vi "Project TMP36.vi"() -> ()   [LabVIEW 2023]
uses:
  <vilib>/MakerHub/LINX/Public/Peripherals/PWM/PWM Set Duty Cycle 1 Chan.vi
  <vilib>/MakerHub/LINX/Public/Utilities/Open Serial.vi
  <vilib>/addons/control/pid/pid.llb/PID (DBL).vi
  <vilib>/MakerHub/LINX/Public/Peripherals/PWM/PWM Set Duty Cycle N Chans.vi
  <vilib>/MakerHub/LINX/Public/Sensors/Temperature/TMP3x/TMP36.vi
  <vilib>/addons/control/pid/NI_PID_pid.lvlib
  <vilib>/MakerHub/LINX/LMH-LINX.lvlib
  <vilib>/MakerHub/LINX/Public/Sensors/Temperature/TMP3x/TMP3x.lvlib
panel:
  in  "LowPass Filter\nTf = x Ts":dbl
  out "u":dbl format="%_2f V"
  out "Tout":dbl format="%_4f °C"
  in  "Ts":dbl
  out "Waveform Chart":dbl(graph)
  in  "Initial Value":dbl
  in  "Set Point":dbl
  in  "Stop Button":bool
  in  "PID Controller":cluster{"Kp":dbl, "Ti":dbl, "Td":dbl}
  # "Temperature"
  # "Time"
  # "PID Control"
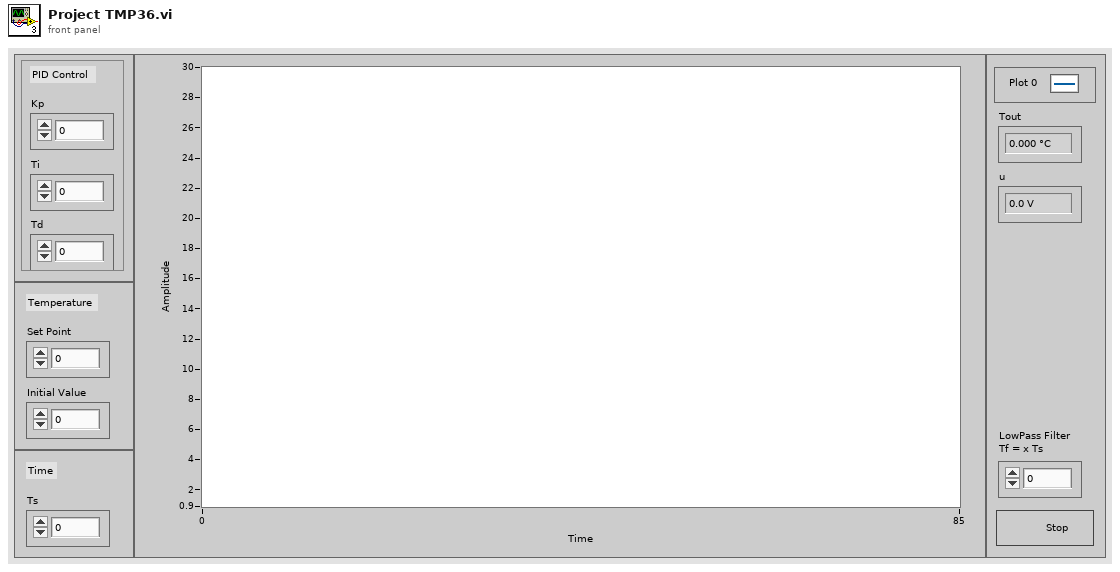
[diagram p1: front panel]
types:
  T1 = typedef "LMH-LINX.lvlib/LINX Ref.ctl" = cluster{"IO":T2, "Interface":T3, "LINX Device Config":T4}
  T2 = typedef "LMH-LINX.lvlib/Platform.ctl" = enum16{"Remote", "Local"}
  T3 = typedef "LMH-LINX.lvlib/Interface.ctl" = enum16{"Serial", "TCP"}
  T4 = typedef "LMH-LINX.lvlib/Device.lvlib/LINX Device Config.ctl" = cluster{"Interface":T3, "COM Port":refnum<visa-resource-name>, "TCP Configuration":T5, "Device Family":u8, "Device ID":u8, "Device Name":string, "TCP Ref":refnum<k5>, "Channels":T6}
  T5 = typedef "LMH-LINX.lvlib/Device.lvlib/TCP Config.ctl" = cluster{"IP Address":string, "Port":u16}
  T6 = typedef "LMH-LINX.lvlib/Channels.ctl" = cluster{"DI":u8[], "DO":u8[], "AI":u8[], "AO":u8[], "PWM":u8[], "QE":u8[], "UART":u8[], "I2C 2":u8[], "SPI":u8[], "CAN":u8[], "Servo":u8[], "AI Ref (V)":dbl, "AI Resolution (Bits)":u8, "AO Ref (V)":dbl, "AO Resolution (Bits)":u8}
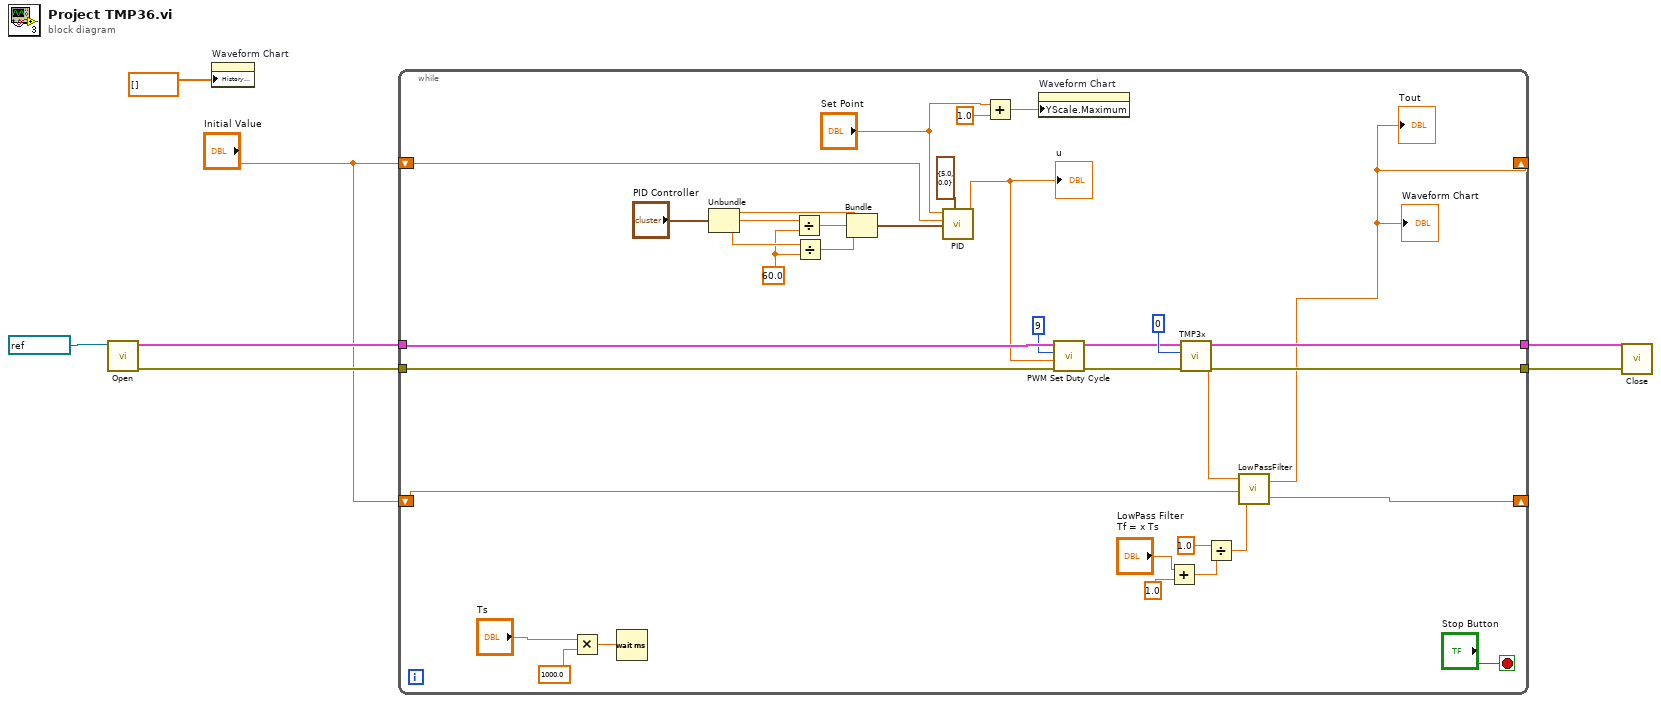
[diagram p0: block diagram]
diagram:
  n1 = call-poly <vilib>:"Open.vi"("Serial Port"=refnum<visa-resource-name> "COM9") -> ("Error Out"=w4:errorcluster, "LINX Resource"=w5:T1)  [unwired: 8 in, 1 out]
  n2 = property on="Waveform Chart" class="WFChart (strict)"("History Data"=dbl[] []) -> ()  [unwired: 2 in, 2 out]
  n3 = while {
    shift-right: [w22] -> _
    shift-left: "Initial Value" -> [w31]
    tunnel: w5 -> [w14]
    tunnel: w4 -> [w11]
    tunnel: [w26] -> w3
    tunnel: [w25] -> w2
    shift-right: [w21] -> _
    shift-left: "Initial Value" -> [w20]
    stop <- "Stop Button" stop-if-true
    w38 = 60.0 ("y")
    n4 = Multiply(x="Ts", y=1000.0) -> (x*y=w32:dbl)
    n5 = Wait (ms)(milliseconds to wait=w32) -> ()  [unwired: 1 out]
    n6 = Unbundle("PID Controller") -> ("Kp"=w36:dbl, "Ti"=w40:dbl, "Td"=w39:dbl)
    n7 = Divide(x=w40, y=w38) -> (x/y=w37:dbl)
    n8 = Divide(x=w39, y=w38) -> (x/y=w35:dbl)
    n9 = Bundle("Kp"=w36, w37, w35) -> (w34:cluster{"Kp":dbl, dbl, dbl})  [unwired: 1 in]
    n10 = call-poly <vilib>:"PID.vi"("output range"=cluster{"output high":dbl, "output low":dbl} {"output high"=5.0, "output low"=0.0}, "PID gains"=w34, "process variable"=w31, "setpoint"="Set Point") -> ("output"=w12:dbl)  [unwired: 6 in, 1 out]
    "u" <- w12
    n11 = Add(x="Set Point", y=1.0) -> (x+y=w28:dbl)
    n12 = property on="Waveform Chart" class="WFChart (strict)"("YScale.Maximum"=w28) -> ()  [unwired: 2 in, 2 out]
    n13 = call-poly <vilib>:"PWM Set Duty Cycle.vi"("Error In"=w11, "Duty Cycle (0-1)"=w12, "PWM Channel"=u8 9 ("AO Channel"), "LINX Resource"=w14) -> ("Error Out"=w9:errorcluster, "LINX Resource"=w10:T1)  [unwired: 6 in]
    n14 = Add(x="LowPass Filter\nTf = x Ts", y=1.0) -> (x+y=w18:dbl)
    n15 = call-poly <vilib>:"TMP3x.vi"("Error In"=w9, "Analog Channel"=u8 0, "LINX Resource"=w10) -> ("Error Out"=w25:errorcluster, "Temp C"=w23:dbl, "LINX Resource"=w26:T1)  [unwired: 6 in]
    n16 = Divide(x=1.0, y=w18) -> (x/y=w15:dbl)
    n17 = call "LowPassFilter.vi"("a"=w15, "yf_prev"=w20, "Tout"=w23) -> ("yf"=w21:dbl, "Tout"=w22:dbl)
    "Waveform Chart" <- w22
    "Tout" <- w22
  }
  n18 = call <vilib>:"Close.vi"("Error In"=w2, "LINX Resource"=w3) -> ()  [unwired: 9 in, 1 out]
